vi "Measurement UI.vi"() -> ()   [LabVIEW 2021, in "Voltage Measurement UI.lvlib"]
uses:
  Voltage Measurement UI.lvlib
  18ef9ac0-ade5-4170-909d-7b230aa6d920.vi
  8290f6cc-02e8-445f-8149-869ff7b03f58.vi
  d72fa500-25b1-4ad4-9a1d-7fe7985d95b9.vi
  c4fed1c9-c021-42fb-90b5-808227222ec8.vi
  822924f3-0171-4e7b-bb5a-3d0262689fc6.vi
  29f62dd2-98c2-4346-a99b-76acf601621e.vi
  e96a8efb-ec4b-4fe5-b7d1-140797539d08.vi
  18ef9ac0-ade5-4170-909d-7b230aa6d920.vi/331b549c-fcf8-43d9-8a1e-5b3c0091a99c.vi
  8290f6cc-02e8-445f-8149-869ff7b03f58.vi/331b549c-fcf8-43d9-8a1e-5b3c0091a99c.vi
  d72fa500-25b1-4ad4-9a1d-7fe7985d95b9.vi/331b549c-fcf8-43d9-8a1e-5b3c0091a99c.vi
  c4fed1c9-c021-42fb-90b5-808227222ec8.vi/331b549c-fcf8-43d9-8a1e-5b3c0091a99c.vi
  822924f3-0171-4e7b-bb5a-3d0262689fc6.vi/6651a77e-856e-4bcd-af5a-c0c13b264cc1.vi
  29f62dd2-98c2-4346-a99b-76acf601621e.vi/6651a77e-856e-4bcd-af5a-c0c13b264cc1.vi
  e96a8efb-ec4b-4fe5-b7d1-140797539d08.vi/6651a77e-856e-4bcd-af5a-c0c13b264cc1.vi
  <vilib>/JDP Science/JSONtext/Variant to JSON Text.vi
  <vilib>/JDP Science/JSONtext/JSON text to Variant.vi
  <vilib>/JDP Science/JSONtext/LVClass Serializer/JSONtext LVClass Serializer.lvclass
panel:
  out "Measurement from SMU Str":string
  in  "Current Config Str":string
  in  "Voltage Config Str":string
  out "Waveform Graph":dbl[](graph)
  out "Measurement from SMU":T1
  in  "Current Config":T2={"Current Limit"=0.01, "Current Limit Range"=0.01} {"Current Limit Range" format="%.3p"; "Current Limit" format="%.3p"}
  in  "Voltage Config":T3={"Voltage Level"=2.0, "Voltage Level Range"=6.0} {"Voltage Level Range" format="%.5p"; "Voltage Level" format="%.5p"}
  out "Signal Out of Range":bool
  out "Measurement":dbl format="%.6p"
  in  "Resolution in Digits":dbl(ring)=5.5 items=["3 1/2"=3.5, "4 1/2"=4.5, "5 1/2"=5.5, "6 1/2"=6.5, "7 1/2"=7.5]
  in  "Range":dbl=10.0 format="%.2f"
  in  "Device Name Pin":string(combo)="Dev1" caption="Device Name"
  in  "Vin SMU Pin":string(combo)="Dev1" caption="Vin SMU"
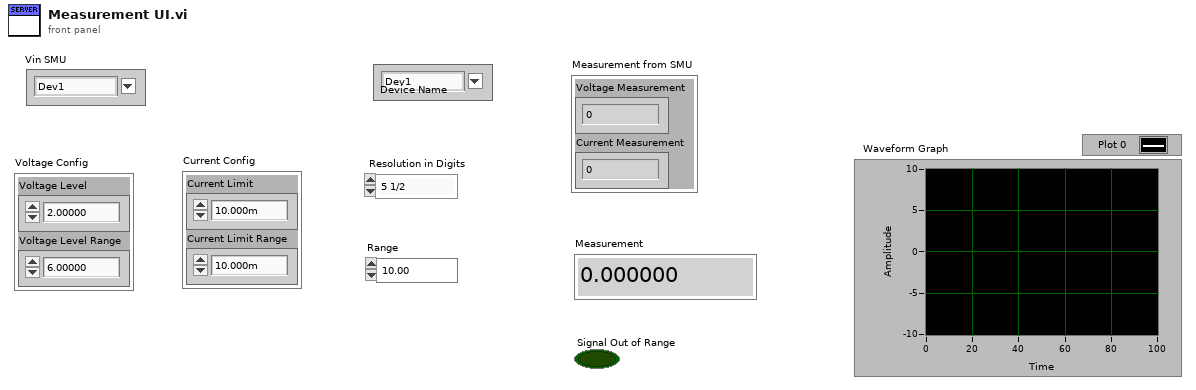
[diagram p1: front panel]
types:
  T1 = cluster{"Voltage Measurement":dbl, "Current Measurement":dbl}
  T2 = cluster{"Current Limit":dbl, "Current Limit Range":dbl}
  T3 = cluster{"Voltage Level":dbl, "Voltage Level Range":dbl}
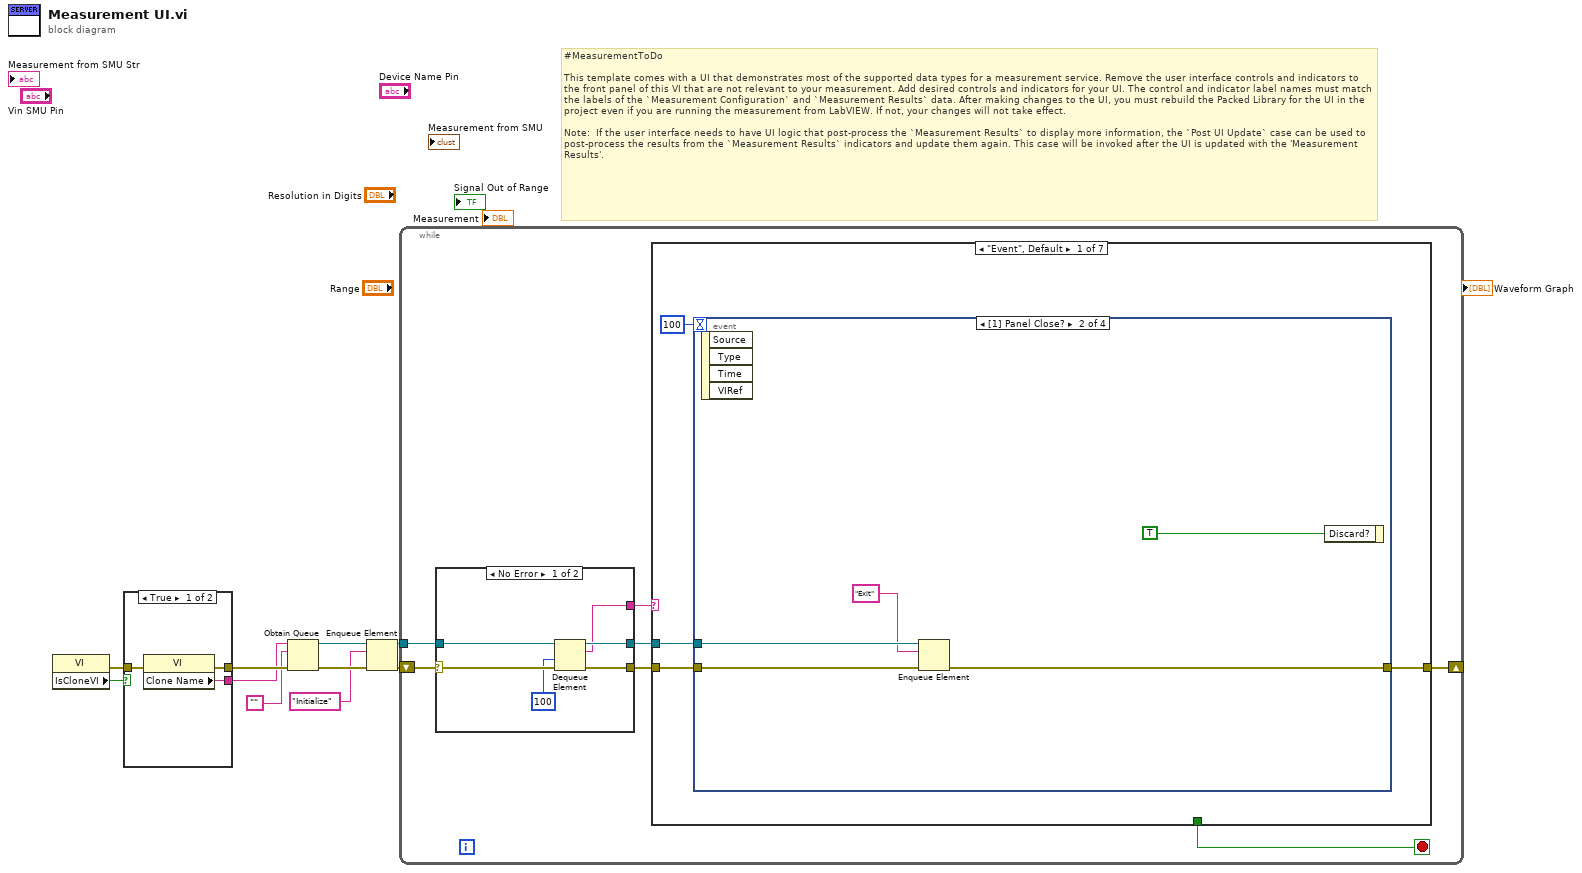
[diagram p0: block diagram]
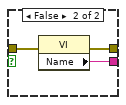
[diagram p2: hidden frame]
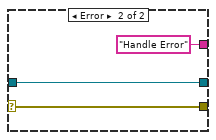
[diagram p3: hidden frame]
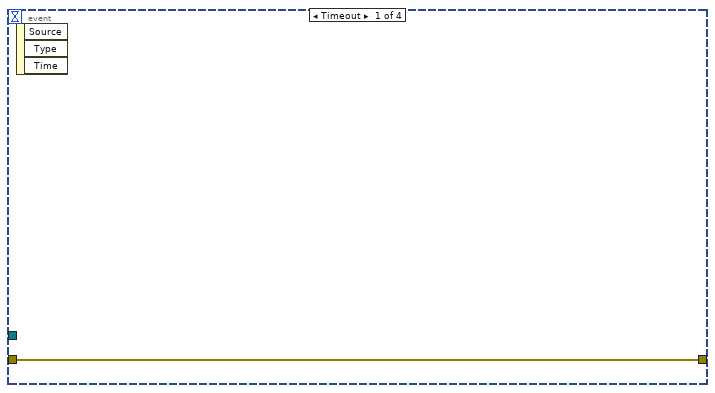
[diagram p4: hidden frame]
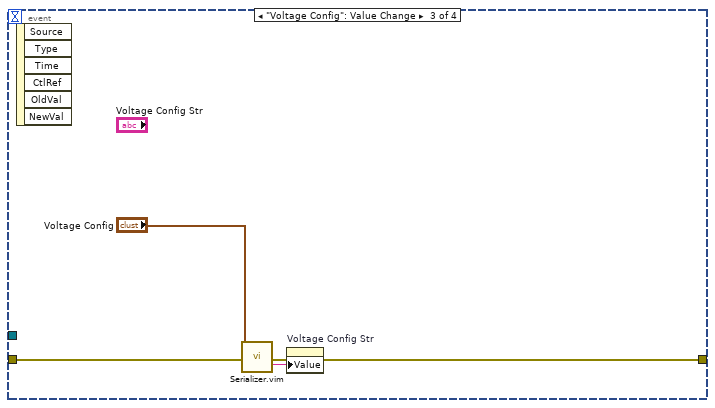
[diagram p5: hidden frame]
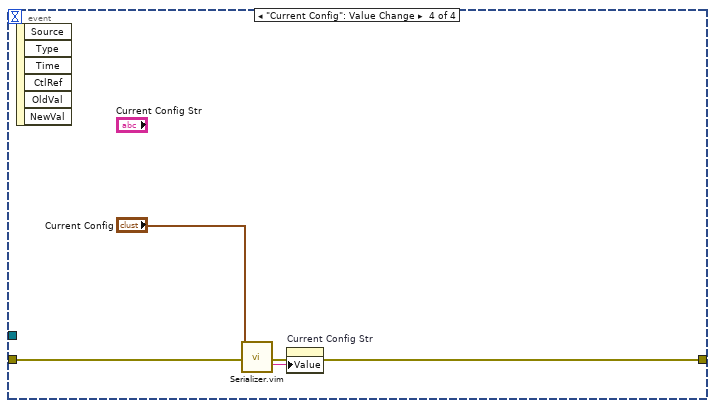
[diagram p6: hidden frame]
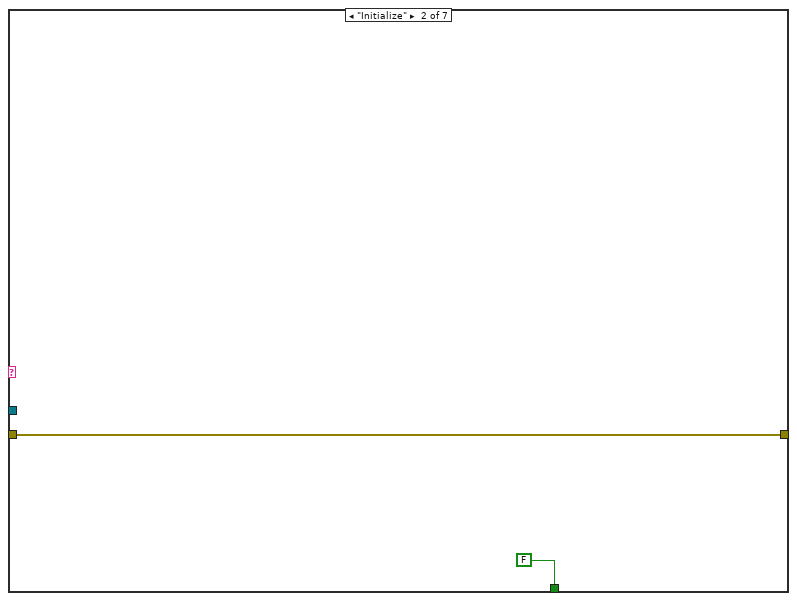
[diagram p7: hidden frame]
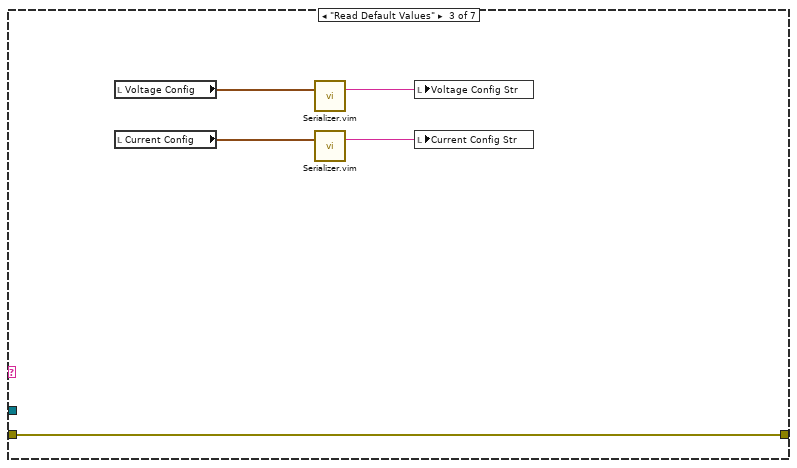
[diagram p8: hidden frame]
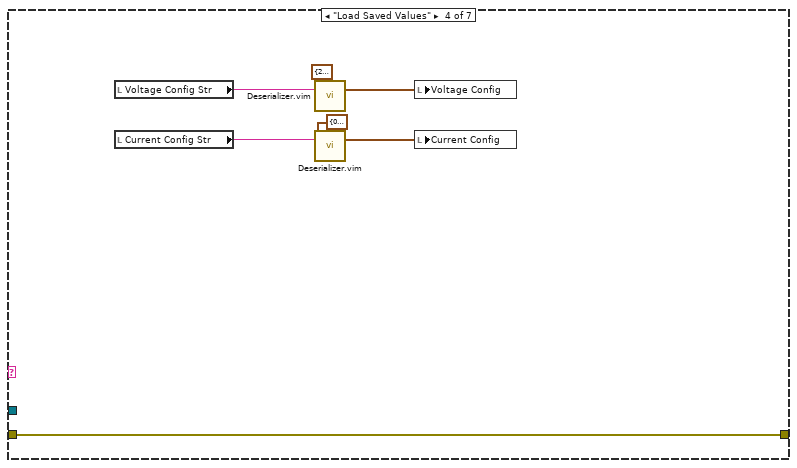
[diagram p9: hidden frame]
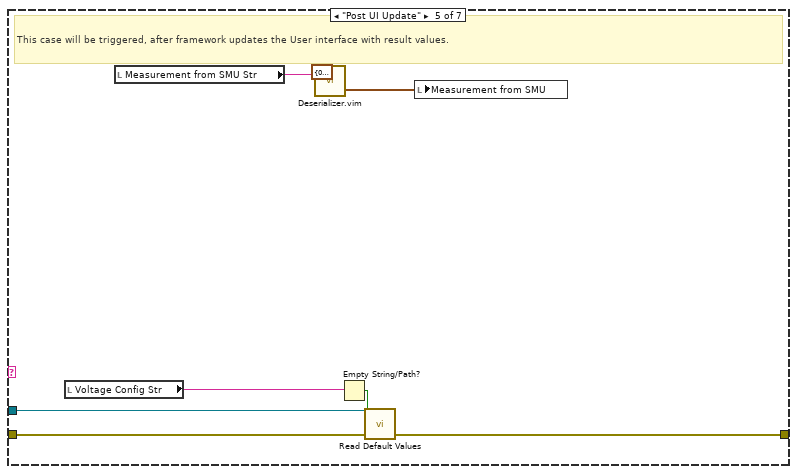
[diagram p10: hidden frame]
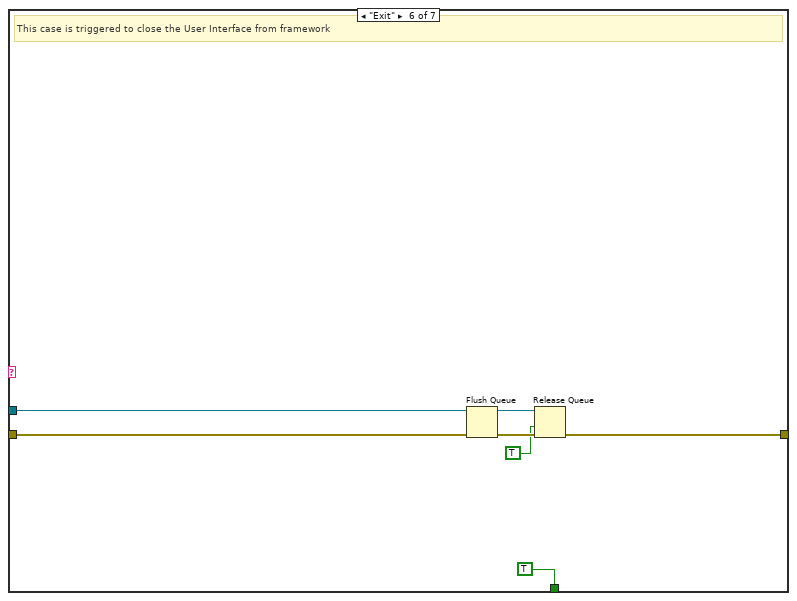
[diagram p11: hidden frame]
diagram:
  # "#MeasurementToDo  \n\nThis template comes with a UI that demonstrates most of the supported data types for a measurement service. Remove the user interface controls and indicators to the front panel of this VI that are not relevant to your measurement. Add desired controls and indicators for your UI. The control and indicator label names must match the labels of the `Measurement Configuration` and `Measurement Results` data. After making changes to the UI, you must rebuild the Packed Library for the UI in the project even if you are running the measurement from LabVIEW. If not, your changes will not take effect.\n\nNote:  If the user interface needs to have UI logic that post-process the `Measurement Results` to display more information, the `Post UI Update` case can be used to post-process the results from the `Measurement Results` indicators and update them again. This case will be invoked after the UI is updated with the 'Measurement Results'."
  n1 = property class="VI"() -> (error out=w1:errorcluster, "IsCloneVI"=w2:bool)  [unwired: 2 in, 1 out]
  n2 = case shown="True" w2 {
    tunnel: [w13 w16] -> w10
    tunnel: [w12 w15] -> w9
    tunnel: w1 -> [w11 w14]
    frame True {
      n3 = property class="VI"(error in=w11) -> (error out=w13:errorcluster, "Clone Name"=w12:string)  [unwired: 1 in, 1 out]
    }
    frame False {
      n4 = property class="VI"(error in=w14) -> (error out=w16:errorcluster, "Name"=w15:string)  [unwired: 1 in, 1 out]
    }
  }
  n5 = Obtain Queue(name (unnamed)=w9, element data type="", error in (no error)=w10) -> (queue out=w6:refnum<queue>, error out=w8:errorcluster)  [unwired: 2 in, 1 out]
  n6 = Enqueue Element(queue=w6, element="Initialize", error in (no error)=w8) -> (queue out=w5:refnum<queue>, error out=w7:errorcluster)  [unwired: 1 in, 1 out]
  n7 = while {
    shift-right: [w18] -> _
    shift-left: w7 -> [w23]
    tunnel: w5 -> [w21]
    stop <- w17 stop-if-true
    n8 = case shown="No Error" w23 {
      selector: w23 -> [w29 w32]
      tunnel: [w28 w32] -> w22
      tunnel: w21 -> [w27 w31]
      tunnel: [w26 w31] -> w20
      tunnel: [w25 "Handle Error"] -> w19
      frame No Error {
        n9 = Dequeue Element(queue=w27, timeout in ms (-1)=100, error in (no error)=w29) -> (queue out=w26:refnum<queue>, element=w25:string, error out=w28:errorcluster)  [unwired: 1 out]
      }
      frame Error {
      }
    }
    n10 = case shown="\"Event\", Default" w19 {
      tunnel: w22 -> [w35 w52 w53 w58 w70 w79 w80]
      tunnel: w20 -> [w33 _ _ _ w69 w77 _]
      tunnel: [w36 w52 w53 w58 w68 w74 w80] -> w18
      tunnel: [_ FALSE _ _ _ TRUE _] -> w17
      frame "Event", Default {
        n11 = event shown="[1] Panel Close?" {
          selector: _ -> [_ _ _ _]
          dyn-events: _ -> [_ _ _ _]
          timeout: 100 -> [_ _ _ _]
          tunnel: [w37 w40 w44 w48] -> w36
          tunnel: w35 -> [w37 w41 w43 w47]
          tunnel: w33 -> [_ w39 _ _]
          event Timeout {
            n12 = event-data() -> ()  [unwired: 1 in, 3 out]
          }
          event Panel Close? {
            n13 = event-data() -> ()  [unwired: 1 in, 4 out]
            n14 = Enqueue Element(queue=w39, element="Exit", error in (no error)=w41) -> (error out=w40:errorcluster)  [unwired: 1 in, 2 out]
            n15 = event-data("Discard?"=TRUE) -> ()  [unwired: 1 in, 1 out]
          }
          event "Voltage Config": Value Change {
            n16 = event-data() -> ()  [unwired: 1 in, 6 out]
            n17 = call "Serializer.vim"("Anything"="Voltage Config", "error in"=w43) -> ("Flattened Data"=w45:string, "error out"=w44:errorcluster)  [unwired: 12 in]
            n18 = property on="Voltage Config Str" class="Str"("Value"=w45) -> ()  [unwired: 2 in, 2 out]
          }
          event "Current Config": Value Change {
            n19 = event-data() -> ()  [unwired: 1 in, 6 out]
            n20 = call "Serializer.vim"("Anything"="Current Config", "error in"=w47) -> ("Flattened Data"=w49:string, "error out"=w48:errorcluster)  [unwired: 12 in]
            n21 = property on="Current Config Str" class="Str"("Value"=w49) -> ()  [unwired: 2 in, 2 out]
          }
        }
      }
      frame "Initialize" {
      }
      frame "Read Default Values" {
        n22 = local read "Voltage Config"() -> (w57:T3)
        n23 = local read "Current Config"() -> (w55:T2)
        n24 = call "Serializer.vim"("Anything"=w57) -> ("Flattened Data"=w56:string)  [unwired: 13 in, 1 out]
        n25 = call "Serializer.vim"("Anything"=w55) -> ("Flattened Data"=w54:string)  [unwired: 13 in, 1 out]
        n26 = local write "Voltage Config Str"(w56) -> ()
        n27 = local write "Current Config Str"(w54) -> ()
      }
      frame "Load Saved Values" {
        n28 = local read "Voltage Config Str"() -> (w64:string)
        n29 = local read "Current Config Str"() -> (w61:string)
        n30 = call "Deserializer.vim"("Flattened Data"=w64, "Data Type"=T3 {"Voltage Level"=2.0, "Voltage Level Range"=6.0} ("Voltage Config")) -> ("Data Out"=w63:T3)  [unwired: 12 in, 1 out]
        n31 = call "Deserializer.vim"("Flattened Data"=w61, "Data Type"=T2 {"Current Limit"=0.01, "Current Limit Range"=0.01} ("Current Config")) -> ("Data Out"=w60:T2)  [unwired: 12 in, 1 out]
        n32 = local write "Voltage Config"(w63) -> ()
        n33 = local write "Current Config"(w60) -> ()
      }
      frame "Post UI Update" {
        # "This case will be triggered, after framework updates the User interface with result values."
        n34 = local read "Voltage Config Str"() -> (w72:string)
        n35 = local read "Measurement from SMU Str"() -> (w67:string)
        n36 = call "Deserializer.vim"("Flattened Data"=w67, "Data Type"=T1 {"Voltage Measurement"=0.0, "Current Measurement"=0.0} ("Measurement from SMU")) -> ("Data Out"=w66:T1)  [unwired: 12 in, 1 out]
        n37 = Empty String/Path?(string/path=w72) -> (empty?=w71:bool)
        n38 = call "Read Default Values.vi"("Queue Ref"=w69, "Empty string?"=w71, "error in"=w70) -> ("error out"=w68:errorcluster)  [unwired: 12 in]
        n39 = local write "Measurement from SMU"(w66) -> ()
      }
      frame "Exit" {
        # "This case is triggered to close the User Interface from framework"
        n40 = Flush Queue(queue=w77, error in (no error)=w79) -> (queue out=w76:refnum<queue>, error out=w75:errorcluster)  [unwired: 1 out]
        n41 = Release Queue(queue=w76, force destroy? (F)=TRUE, error in (no error)=w75) -> (error out=w74:errorcluster)  [unwired: 2 out]
      }
      frame "Handle Error" {
      }
    }
  }
